vi "Init.vi"(8 "error in (no error)":errorcluster, 11 "UI Actor in":refnum<class "UI Actor.lvclass">) -> (0 "error out":errorcluster, 3 "UI Actor out":refnum<class "UI Actor.lvclass">)   [LabVIEW 2019, in "UI Actor.lvlib" / "UI Actor.lvclass"]
uses:
  UI Actor.lvclass
  C:/Program Files/National Instruments/LabVIEW 2019/vi.lib/ActorFramework/Actor/Actor.lvclass
  UI Actor.lvclass/UI Actor.ctl
  Actor_C_MXN/Actor_C_MXN.lvclass
  Actor_C_MXN/Actor_C_MXN.lvclass/Actor_C_MXN.ctl
  Actor_USD/Actor_USD.lvclass
  Actor_USD/Actor_USD.lvclass/Actor_USD.ctl
  Read Monedas.vi
  Read Sub Panel Coins.vi
  <vilib>/ActorFramework/Actor/Actor.lvclass
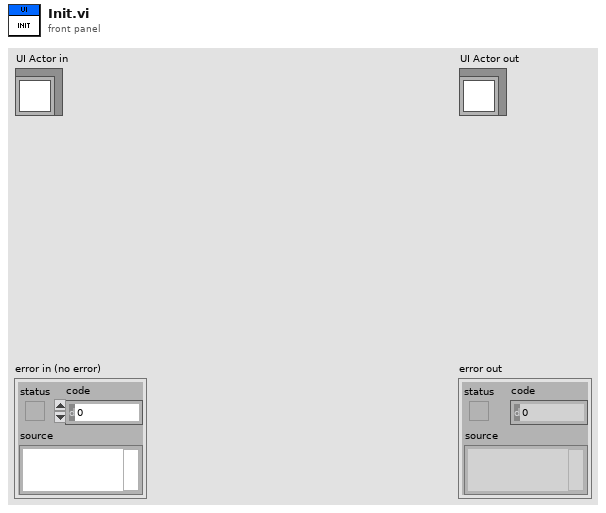
[diagram p1: front panel]
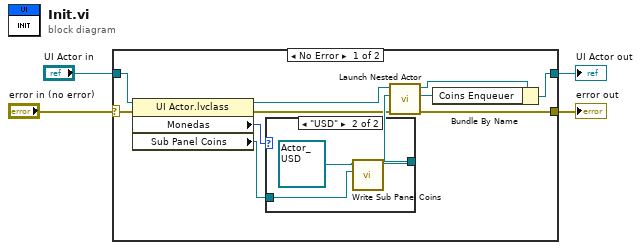
[diagram p0: block diagram]
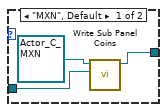
[diagram p2: hidden frame]
diagram:
  n1 = case shown="No Error" "error in (no error)" {
    selector: "error in (no error)" -> [w9 w23]
    tunnel: [w13 w23] -> w3
    tunnel: [w7 w22] -> w1
    tunnel: "UI Actor in" -> [w15 w22]
    frame No Error {
      n2 = property class="UI Actor.lvclass"(reference=w15, error in=w9) -> (reference out=w11:refnum<class "UI Actor.lvclass">, error out=w8:errorcluster, "Monedas"=w14:enum16{"MXN", "USD"}, "Sub Panel Coins"=w5:refnum<vi>)
      n3 = case shown="\"USD\"" w14 {
        tunnel: [w17 w20] -> w12
        tunnel: w5 -> [w16 w19]
        frame "MXN", Default {
          n4 = call "Write Sub Panel Coins.vi"("Sub Panel Coins"=w16, "Actor_C_MXN in"=refnum<class "Actor_C_MXN.lvclass"> refnum ("Actor_C_MXN.lvlib:Actor_C_MXN.lvclass")) -> ("Actor_C_MXN out"=w17:refnum<class "Actor_C_MXN.lvclass">)  [unwired: 8 in, 1 out]
        }
        frame "USD" {
          n5 = call "Write Sub Panel Coins.vi"("Sub Panel Coins"=w19, "Actor_USD in"=refnum<class "Actor_USD.lvclass"> refnum ("Actor_USD.lvlib:Actor_USD.lvclass")) -> ("Actor_USD out"=w20:refnum<class "Actor_USD.lvclass">)  [unwired: 8 in, 1 out]
        }
      }
      n6 = call <vilib>:"Launch Nested Actor.vi"("error in (no error)"=w8, "Nested Actor"=w12, "Caller Actor in"=w11) -> ("error out"=w13:errorcluster, "Nested Actor's Enqueuer"=w6:refnum<class "Message Enqueuer.lvclass">, "Caller Actor out"=w10:refnum<class "UI Actor.lvclass">)  [unwired: 6 in]
      n7 = Bundle By Name(cluster=w10, "Coins Enqueuer"=w6) -> (w7:refnum<class "UI Actor.lvclass">)
    }
    frame Error {
    }
  }
  "error out" <- w3
  "UI Actor out" <- w1
